vi "freq_response_scan_ref_aux.vi"(10 "Testing":i32, 11 "Trace controls in":T1[](array[typedef])) -> (3 "Trace controls out":T1[](array[typedef]))   [LabVIEW 2012]
uses:
  Trace controls.ctl
  probe_point.ctl
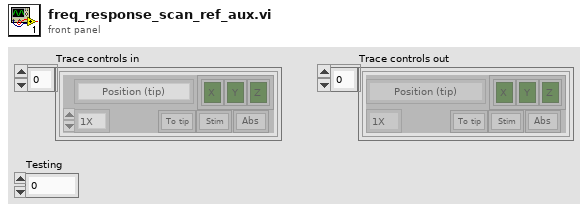
[diagram p1: front panel]
types:
  T1 = typedef "Trace controls.ctl" = cluster{"+ stim":bool, "Relative":bool, "Scale":enum16{"1X", "10X", "100X", "1KX", "10KX"}, "Probe point":T2, "XYZ selector":cluster{"Boolean":bool, "Boolean 2":bool, "Boolean 3":bool}, "To tip":bool}
  T2 = typedef "probe_point.ctl" = enum16{"Position (tip)", "Position (RCM)", "Null pos (tip)", "Null pos (RCM)", "V limiter (tip)", "V Limiter (RCM)", "Goal (tip)", "Goal (RCM)", "Link pos 0", "Link pos 1", "KF link pos 0", "KF link pos 1", "Link rate 0", "Link rate 1", "Link residue 0", "Link residue 1", "Link goal 0", "Link goal 1", "Rate limit 0", "Rate limit 1", "Link error 0", "Link error 1", "Controller 0", "Controller 1", "Output 0", "Output 1", "Drive 0", "Drive 1", "Stimulus 0", "Stimulus 1", "Trace data 0", "Trace data 1", "Analog data 0", "Analog data 1", "Status flags", "Light 0", "Light 1", "Light 2", "Light 3", "Light 4", "Light 5", "Goal origin", "Goal rotation 0", "Goal rotation 1", "Goal rotation 2", "Output origin", "Output rotation 0", "Output rotation 1", "Output rotation 2", "Handle origin", "Handle rotation 0", "Handle rotation 1", "Handle rotation 2", "Handle position", "Handle velocity", "Handle acceleration", "Handle angles", "Handle angle rates", "Handle pos residue", "Handle angle residue", "Trace length"}
  T3 = cluster{"Boolean":bool, "Boolean 2":bool, "Boolean 3":bool}
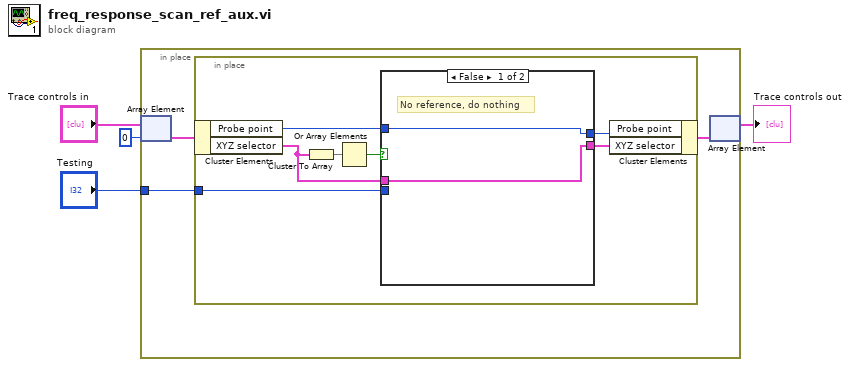
[diagram p0: block diagram]
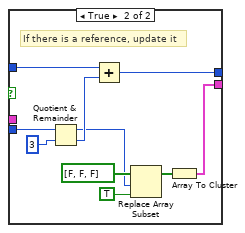
[diagram p2: hidden frame]
diagram:
  n1 = in-place {
    in-place-border: "Testing" -> [w5]
    n2 = in-place-array #1("Trace controls in", 0) -> (w7:T1)
    n3 = in-place {
      in-place-border: w5 -> [w14]
      n4 = in-place-cluster #2(w7) -> ("Probe point"=w12:T2, "XYZ selector"=w8:T3)
      n5 = Cluster To Array(cluster=w8) -> (array=w10:bool[])
      n6 = Or Array Elements(Boolean array=w10) -> (logical OR=w9:bool)
      n7 = case shown="False" w9 {
        tunnel: w14 -> [_ w26]
        tunnel: [w16 w24] -> w13
        tunnel: w12 -> [w16 w23]
        tunnel: [w15 w17] -> w11
        tunnel: w8 -> [w15 _]
        frame False {
          # "No reference, do nothing"
        }
        frame True {
          # "If there is a reference, update it"
          n8 = Quotient & Remainder(x=w26, y=3) -> (x-y*floor(x/y)=w19:i32, floor(x/y)=w22:i32)
          n9 = Add(x=w23, y=w22) -> (x+y=w24:i32)
          n10 = Replace Array Subset(array=bool[] [FALSE, FALSE, FALSE], new element=TRUE, index=w19) -> (w18:bool[])
          n11 = Array To Cluster(array=w18) -> (cluster=w17:cluster{"[0]":bool, "[1]":bool, "[2]":bool})
        }
      }
      n12 = in-place-cluster #2("Probe point"=w13, "XYZ selector"=w11) -> (w6:T1)
    }
    n13 = in-place-array #1(w6) -> (→"Trace controls out":T1[])  [unwired: 1 out]
  }
